vi "flower_watering_reports.vi"(1 "from (0:start)":enum16{"start", "end", "current"}(ring), 2 "Numeric":i32, 3 "Reports filepath":path=path "C:/reports.txt", 4 "access (0:read/write)":enum16{"read/write", "read-only", "write-only"}(ring)) -> ()   [LabVIEW 2021]
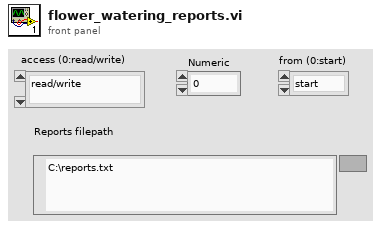
[diagram p1: front panel]
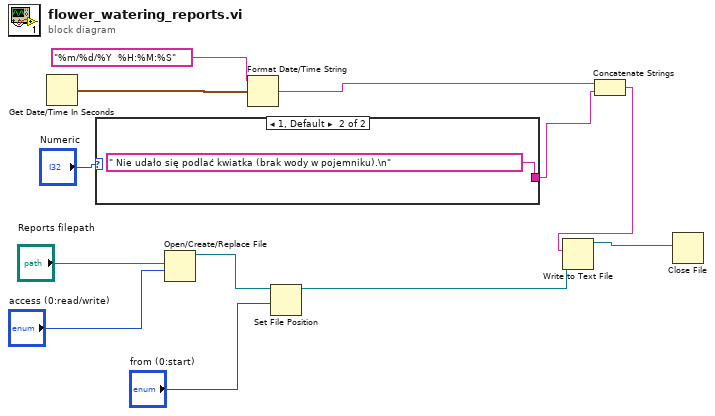
[diagram p0: block diagram]
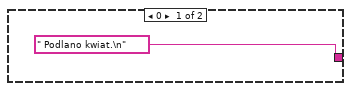
[diagram p2: hidden frame]
diagram:
  n1 = Get Date/Time In Seconds() -> (seconds since 1Jan1904=w8:timestamp)
  n2 = case shown="1, Default" "Numeric" {
    tunnel: [" Podlano kwiat.\n" " Nie udało się podlać kwiatka (brak wody w pojemniku).\n"] -> w5
    frame 0 {
    }
    frame 1, Default {
    }
  }
  n3 = Open/Create/Replace File(file path (use dialog)="Reports filepath", access (0:read/write)="access (0:read/write)") -> (refnum out=w11:refnum<file>)  [unwired: 4 in, 2 out]
  n4 = Format Date/Time String(time format string (%c)="%m/%d/%Y  %H:%M:%S", seconds (now)=w8) -> (date/time string=w6:string)  [unwired: 1 in]
  n5 = Set File Position(refnum=w11, from (0:start)="from (0:start)") -> (refnum out=w10:refnum<file>)  [unwired: 2 in, 1 out]
  n6 = Concatenate Strings(w6, w5) -> (w4:string)
  n7 = Write to Text File(file (use dialog)=w10, text=w4) -> (refnum out=w9:refnum<file>)  [unwired: 2 in, 2 out]
  n8 = Close File(refnum=w9) -> ()  [unwired: 1 in, 2 out]
